vi "Timer With Pause.vi"(7 "Timer Action":T1, 8 "error in (no error)":errorcluster, 10 "Target Time":dbl) -> (0 "error out":errorcluster, 2 "Elapsed Time":dbl format="%.2g", 3 "Done?":bool)   [LabVIEW 2010]
doc: "Use this template to build a VI to use as a subVI."
uses:
  Controls/Timer Actions ENUM_TDef.ctl
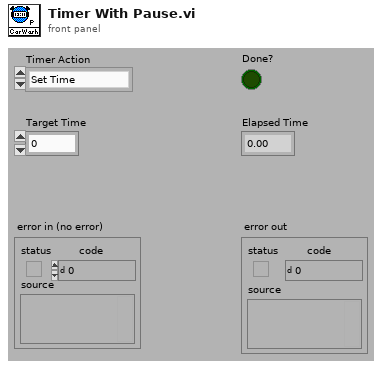
[diagram p1: front panel]
types:
  T1 = typedef "Timer Actions ENUM_TDef.ctl" = enum16{"Set Time", "Get Time", "Pause Time", "Resume Time"}
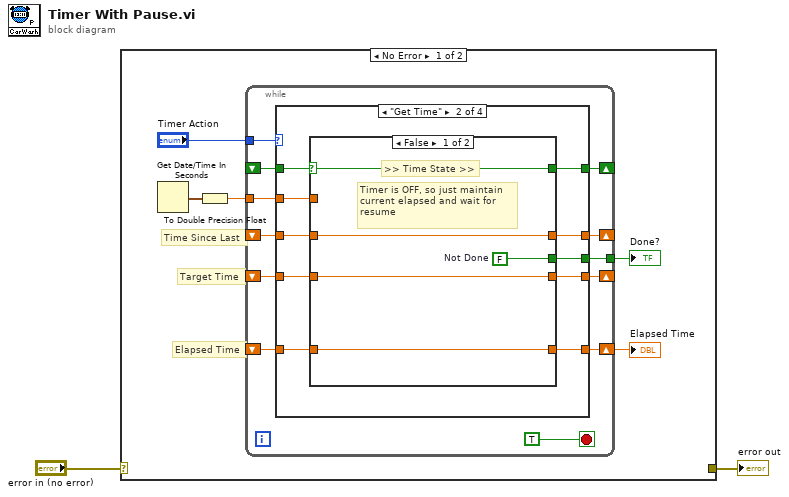
[diagram p0: block diagram]
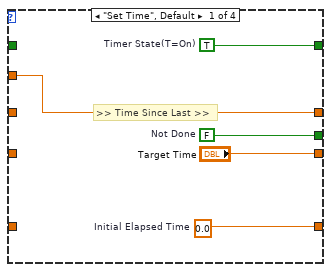
[diagram p2: hidden frame]
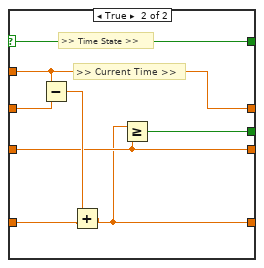
[diagram p3: hidden frame]
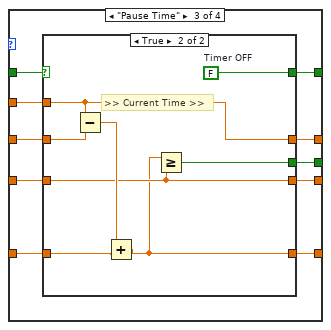
[diagram p4: hidden frame]
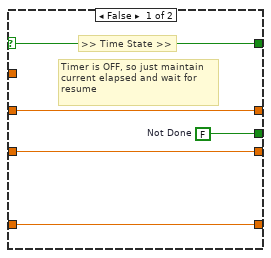
[diagram p5: hidden frame]
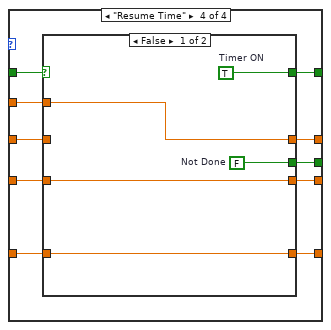
[diagram p6: hidden frame]
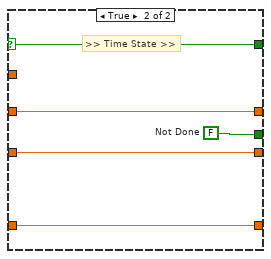
[diagram p7: hidden frame]
diagram:
  n1 = case shown="No Error" "error in (no error)" {
    selector: "error in (no error)" -> [_ w91]
    tunnel: [_ w91] -> w1
    frame No Error {
      # "Elapsed Time"
      # "Target Time"
      # "Time Since Last"
      n2 = Get Date/Time In Seconds() -> (seconds since 1Jan1904=w7:timestamp)
      n3 = To Double Precision Float(number=w7) -> (double precision float=w6:dbl)
      n4 = while {
        tunnel: w6 -> [w13]
        shift-right: [w17] -> w4
        shift-left: _ -> [w16]
        tunnel: "Timer Action" -> [w18]
        shift-right: [w15] -> _
        shift-left: _ -> [w14]
        shift-right: [w12] -> _
        shift-left: _ -> [w10]
        shift-right: [w11] -> _
        shift-left: _ -> [w9]
        tunnel: [w8] -> w3
        stop <- TRUE stop-if-true
        n5 = case shown="\"Get Time\"" w18 {
          tunnel: [w24 w31 w55 w78] -> w17
          tunnel: w16 -> [_ w32 w56 w79]
          tunnel: [w23 w27 w52 w75] -> w15
          tunnel: w14 -> [_ w28 w51 w74]
          tunnel: w13 -> [w22 w33 w50 w73]
          tunnel: [w22 w26 w49 w72] -> w12
          tunnel: ["Target Time" w25 w48 w71] -> w11
          tunnel: w10 -> [_ w34 w57 w80]
          tunnel: w9 -> [_ w30 w54 w77]
          tunnel: [w20 w29 w53 w76] -> w8
          frame "Set Time", Default {
            w20 = FALSE  # Not Done
            w23 = TRUE  # Timer State(T=On)
            w24 = 0.0  # Initial Elapsed Time
            # ">> Time Since Last >>"
          }
          frame "Get Time" {
            n6 = case shown="False" w28 {
              selector: w28 -> [w36 w43]
              tunnel: w34 -> [w37 w47]
              tunnel: w33 -> [_ w42]
              tunnel: w32 -> [w39 w46]
              tunnel: [w39 w40] -> w31
              tunnel: w30 -> [w38 w41]
              tunnel: [w35 w44] -> w29
              tunnel: [w36 w43] -> w27
              tunnel: [w37 w42] -> w26
              tunnel: [w38 w41] -> w25
              frame False {
                w35 = FALSE  # Not Done
                # "Timer is OFF, so just maintain\ncurrent elapsed and wait for\nresume"
                # ">> Time State >>"
              }
              frame True {
                # ">> Current Time >>"
                # ">> Time State >>"
                n7 = Subtract(x=w42, y=w47) -> (x-y=w45:dbl)
                n8 = Add(x=w45, y=w46) -> (x+y=w40:dbl)
                n9 = Greater Or Equal?(x=w40, y=w41) -> (x >= y?=w44:bool)
              }
            }
          }
          frame "Pause Time" {
            n10 = case shown="True" w51 {
              selector: w51 -> [w62 _]
              tunnel: w57 -> [w61 w70]
              tunnel: w50 -> [_ w65]
              tunnel: w56 -> [w59 w69]
              tunnel: [w59 w63] -> w55
              tunnel: w54 -> [w60 w64]
              tunnel: [w58 w67] -> w53
              tunnel: [w62 w66] -> w52
              tunnel: [w61 w65] -> w49
              tunnel: [w60 w64] -> w48
              frame False {
                w58 = FALSE  # Not Done
                # "Timer is OFF, so just maintain\ncurrent elapsed and wait for\nresume"
                # ">> Time State >>"
              }
              frame True {
                w66 = FALSE  # Timer OFF
                # ">> Current Time >>"
                n11 = Subtract(x=w65, y=w70) -> (x-y=w68:dbl)
                n12 = Add(x=w68, y=w69) -> (x+y=w63:dbl)
                n13 = Greater Or Equal?(x=w63, y=w64) -> (x >= y?=w67:bool)
              }
            }
          }
          frame "Resume Time" {
            n14 = case shown="False" w74 {
              selector: w74 -> [_ w89]
              tunnel: w80 -> [_ w86]
              tunnel: w73 -> [w81 _]
              tunnel: w79 -> [w84 w88]
              tunnel: [w84 w88] -> w78
              tunnel: w77 -> [w85 w90]
              tunnel: [w83 w87] -> w76
              tunnel: [w82 w89] -> w75
              tunnel: [w81 w86] -> w72
              tunnel: [w85 w90] -> w71
              frame False {
                w82 = TRUE  # Timer ON
                w83 = FALSE  # Not Done
              }
              frame True {
                w87 = FALSE  # Not Done
                # ">> Time State >>"
              }
            }
          }
        }
      }
      "Done?" <- w3
      "Elapsed Time" <- w4
    }
    frame Error {
    }
  }
  "error out" <- w1
